vi "Get FPGA Ref.vi"(11 "FPGAtarget in":refnum<class "FPGATarget.lvclass">) -> (3 "FPGAref":refnum<vi>)   [LabVIEW 2020, in "NI_TargetHelper.lvlib" / "FPGATarget.lvclass"]
uses:
  <vilib>/TargetSupport/NI_TargetHelper/FPGATarget/FPGATarget.lvclass
  <vilib>/TargetSupport/NI_TargetHelper/FPGATarget/FPGATarget.lvclass/FPGATarget.ctl
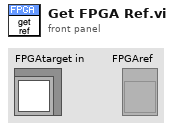
[diagram p1: front panel]
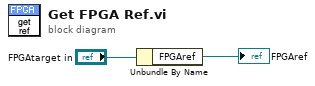
[diagram p0: block diagram]
diagram:
  n1 = Unbundle By Name("FPGAtarget in") -> ("FPGAref"=→"FPGAref":refnum<vi>)
